vi "Drive Base - Update.vi"(8 "error in (no error)":errorcluster, 11 "Drive Base Notifier":T1) -> (0 "error out":errorcluster)   [LabVIEW 2015]
uses:
  Robot Code/Drive Base - Controlled Mode - TypeDef.ctl
  Robot Code/Drive Base Mode.ctl
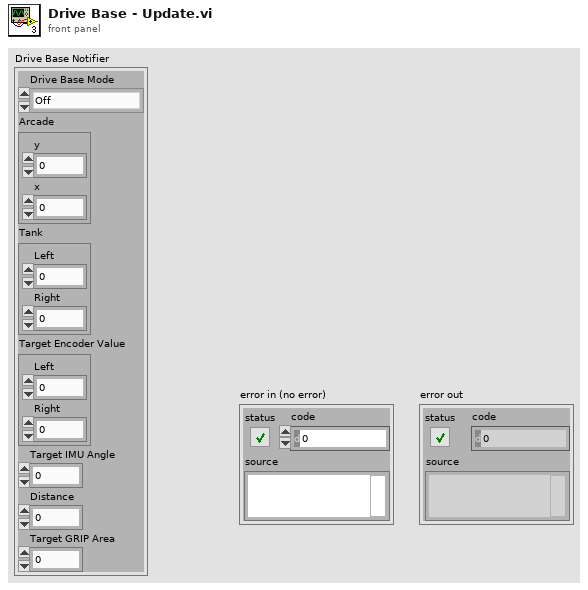
[diagram p1: front panel]
types:
  T1 = typedef "Drive Base - Controlled Mode - TypeDef.ctl" = cluster{"Drive Base Mode":T2, "Arcade":cluster{"y":dbl, "x":dbl}, "Tank":cluster{"Left":dbl, "Right":dbl}, "Target Encoder Value":cluster{"Left":dbl, "Right":dbl}, "Target IMU Angle":dbl, "Distance":dbl, "Target GRIP Area":dbl}
  T2 = typedef "Drive Base Mode.ctl" = enum16{"Off", "Controlled - Arcade", "Controlled - Tank", "Braked", "GRIP", "Encoder", "IMU", "Distance"}
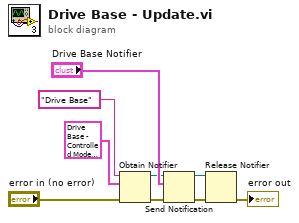
[diagram p0: block diagram]
diagram:
  n1 = Obtain Notifier(name (unnamed)="Drive Base", notification data type=T1 {"Drive Base Mode"=enum."Off", "Arcade"={"y"=0.0, "x"=0.0}, "Tank"={"Left"=0.0, "Right"=0.0}, "Target Encoder Value"={"Left"=0.0, "Right"=0.0}, "Target IMU Angle"=0.0, "Distance"=0.0, "Target GRIP Area"=0.0}, error in (no error)="error in (no error)") -> (notifier out=w4:refnum<notifier>, error out=w5:errorcluster)  [unwired: 1 in, 1 out]
  n2 = Send Notification(notification="Drive Base Notifier", notifier=w4, error in (no error)=w5) -> (notifier out=w7:refnum<notifier>, error out=w6:errorcluster)
  n3 = Release Notifier(notifier=w7, error in (no error)=w6) -> (error out=→"error out":errorcluster)  [unwired: 1 in, 2 out]
